vi "StepperMotorAngleControl.vi"() -> ()   [LabVIEW 2019]
uses:
  <vilib>/Platform/TimedLoop/XDataNode/timing_clust.ctl
  <vilib>/Platform/TimedLoop/XDataNode/nitl_modes.ctl
  <vilib>/Platform/TimedLoop/XDataNode/wakeup.ctl
  <vilib>/Platform/TimedLoop/XDataNode/XDataNode.xnode
  KNRm_ReMi_OS6_436Motor.lvlibp
  <vilib>/Platform/TimedLoop/XDataNode/XDNodeRunTimeDep.lvlib
panel:
  in  "angle":dbl format="%#_13g"
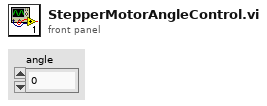
[diagram p1: front panel]
types:
  T1 = typedef "XDNodeRunTimeDep.lvlib/timing_clust.ctl" = cluster{"Expected End [f-1]":u64, "Actual End [f-1]":u64, "Finished Late? [f-1]":bool, "Expected End [i-1]":u64, "Actual End [i-1]":u64, "Finished Late? [i-1]":bool, "Expected Start [i]":u64, "Actual Start [i]":u64, "Expected Start [f]":u64, "Actual Start [f]":u64, "Source Name":string, "Structure Name":string, "Period":i64, "Deadline":i64, "Offset":i64, "Start":i64, "Priority":i32, "Timeout":i32, "Mode":T2, "Wakeup Reason":T3, "Error":errorcluster, "Source Type":string, "Secondary Source Type":string, "Global End Time":u64, "Global Start Time":u64, "Frame Duration":u64, "Iteration Duration":u64, "Assigned CPU":i32, "I/O Scan Engine Mode":u32}
  T2 = typedef "XDNodeRunTimeDep.lvlib/nitl_modes.ctl" = enum32{"No Change", "Process missed periods, maintain original phase", "Discard missed periods, maintain original phase", "Process missed periods, ignore original phase", "Discard missed periods, ignore original phase"}
  T3 = typedef "XDNodeRunTimeDep.lvlib/wakeup.ctl" = enum32{"Normal", "Aborted", "Asynchronous wakeup", "Timing source error", "Timed loop error", "Timeout"}
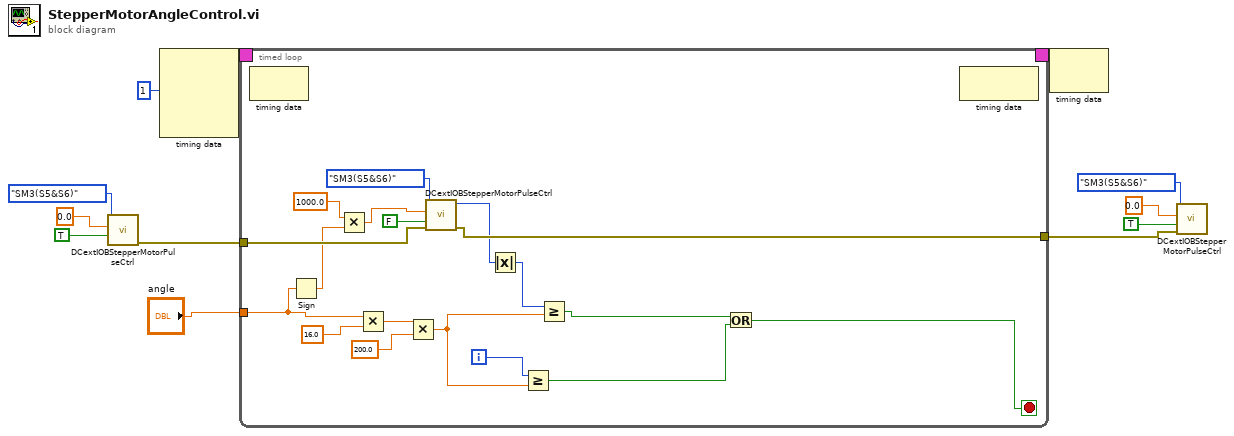
[diagram p0: block diagram]
diagram:
  n1 = call "DCextIOBStepperMotorPulseCtrl.vi"("ResetCounter"=TRUE, "PulseRate&Dir P/S"=0.0, "Port"=enum16{"SM1(S1&S2)", "SM2(S3&S4)", "SM3(S5&S6)"}."SM3(S5&S6)") -> ("error out"=w6:errorcluster)  [unwired: 7 in, 1 out]
  n2 = node-c288(i64 1 ("Period")) -> (w9:T1)  [unwired: 3 in]
  n3 = timed-loop {
    timing: w9 -> [_]
    timing-out: [_] -> w8
    tunnel: w6 -> [w28]
    tunnel: [w27] -> w2
    tunnel: "angle" -> [w23]
    i -> [w15]
    stop <- w17 stop-if-true
    n4 = node-c288() -> ()  [unwired: 1 in, 1 out]
    n5 = Sign(1:w23) -> (0:w22:dbl)
    n6 = Multiply(x=1000.0 ("PulseRate&Dir P/S"), y=w22) -> (x*y=w20:dbl)
    n7 = Multiply(x=w23, y=16.0) -> (x*y=w25:dbl)
    n8 = Multiply(x=w25, y=200.0) -> (x*y=w16:dbl)
    n9 = call "DCextIOBStepperMotorPulseCtrl.vi"("error in"=w28, "ResetCounter"=FALSE, "PulseRate&Dir P/S"=w20, "Port"=enum16{"SM1(S1&S2)", "SM2(S3&S4)", "SM3(S5&S6)"}."SM3(S5&S6)") -> ("error out"=w27:errorcluster, "PulseCounter+/-"=w19:i32)  [unwired: 6 in]
    n10 = Absolute Value(x=w19) -> (abs(x)=w18:i32)
    n11 = Greater Or Equal?(x=w15, y=w16) -> (x >= y?=w13:bool)
    n12 = Greater Or Equal?(x=w18, y=w16) -> (x >= y?=w14:bool)
    n13 = Or(x=w14, y=w13) -> (x .or. y?=w17:bool)
    n14 = node-c288() -> ()  [unwired: 1 in, 1 out]
  }
  n15 = node-c288(w8) -> ()  [unwired: 1 out]
  n16 = call "DCextIOBStepperMotorPulseCtrl.vi"("error in"=w2, "ResetCounter"=TRUE, "PulseRate&Dir P/S"=0.0, "Port"=enum16{"SM1(S1&S2)", "SM2(S3&S4)", "SM3(S5&S6)"}."SM3(S5&S6)") -> ()  [unwired: 6 in, 2 out]
